vi "JYCalibrate.vi"(2 "error in (no error)":errorcluster, 3 "Actual Wavelength":dbl, 4 "JYMONOLib.IJYMonoReqd":refnum<k7>) -> (0 "error out":errorcluster, 1 "JYMONOLib.IJYMonoReqd 2":refnum<k7>)   [LabVIEW 2009]
doc: "JYCalibrate.vi\n\n\nInputs - MonoRefNum - LabView automation refnum for the mono\nUniqueID\n Actual Wavelength Remote - \n Error Cluster\n\nOutputs\n MonoRefNum - the LabView automation refnum for this mono\n is supplied as an output\n\n Error Cluster"
panel:
  out "UseUniqueID":bool
  in  "UniqueID":string
  in  "Mode Select":bool
  # "Local / Front Panel mode"
  # "Remote / Progarm mode"
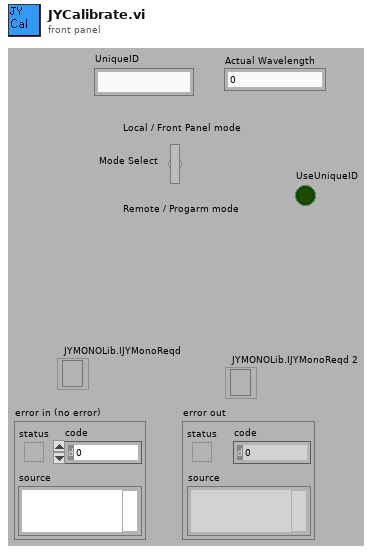
[diagram p1: front panel]
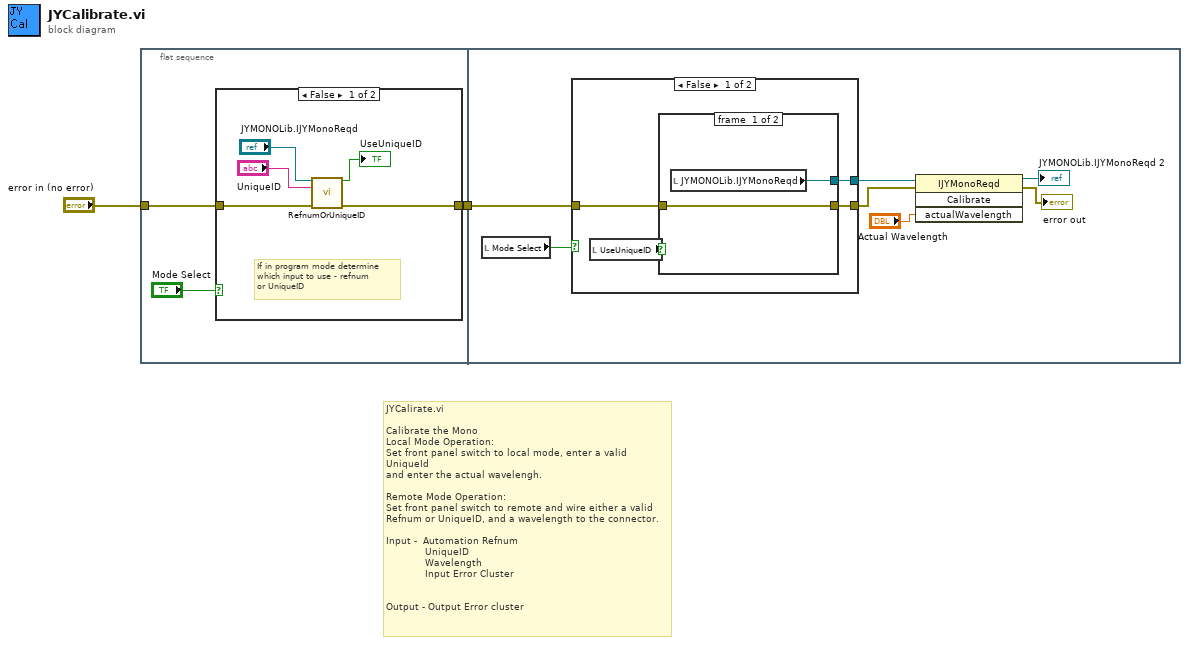
[diagram p0: block diagram]
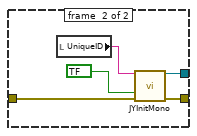
[diagram p3: hidden frame]
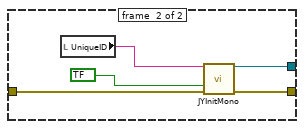
[diagram p4: hidden frame]
diagram:
  # "JYCalirate.vi\n\nCalibrate the Mono\nLocal Mode Operation:\nSet front panel switch to local mode, enter a valid UniqueId\nand enter the actual wavelengh.\n\nRemote Mode Operation:\nSet front panel switch to remote and wire either a valid\nRefnum or UniqueID, and a wavelength to the connector.\n\nInput -  Automation Refnum\n             UniqueID\n             Wavelength\n             Input Error Cluster\n\n\nOutput - Output Error cluster"
  n1 = flat-sequence {
    tunnel: "error in (no error)" -> [w4]
    tunnel: [w3] -> w1
    tunnel: w1 -> [w17]
    frame #0 {
      n2 = case shown="False" "Mode Select" {
        tunnel: w4 -> [w7 w11]
        tunnel: [w6 w11] -> w3
        frame #0 {
          # "If in program mode determine\nwhich input to use - refnum\nor UniqueID"
          n3 = call "RefnumOrUniqueID.vi"("Refnum IN"="JYMONOLib.IJYMonoReqd", "String in"="UniqueID", "error in (no error)"=w7) -> ("UseUniqueID"=→"UseUniqueID":bool, "error out"=w6:errorcluster)  [unwired: 11 out]
        }
        frame #1 {
        }
      }
    }
    frame #1 {
      n4 = local read "Mode Select"() -> (w18:bool)
      n5 = case shown="False" w18 {
        tunnel: w17 -> [w21 w34]
        tunnel: [w20 w31] -> w15
        tunnel: [w19 w30] -> w16
        frame #0 {
          n6 = local read "UseUniqueID"() -> (w22:bool)
          n7 = case shown="True" w22 {
            tunnel: w21 -> [w24 w27]
            tunnel: [w24 w26] -> w20
            tunnel: [w23 w25] -> w19
            frame #0 {
              n8 = local read "JYMONOLib.IJYMonoReqd"() -> (w23:refnum<k7>)
            }
            frame #1 {
              n9 = local read "UniqueID"() -> (w29:string)
              n10 = call "JYInitMono.vi"("Unique ID"=w29, "Force Init"=bool ?, "error in (no error)"=w27) -> ("Mono RefNum out"=w25:refnum<k7>, "error out"=w26:errorcluster)  [unwired: 1 in, 10 out]
            }
          }
        }
        frame #1 {
          n11 = local read "UniqueID"() -> (w33:string)
          n12 = call "JYInitMono.vi"("Unique ID"=w33, "Force Init"=bool ?, "error in (no error)"=w34) -> ("Mono RefNum out"=w30:refnum<k7>, "error out"=w31:errorcluster)  [unwired: 1 in, 10 out]
        }
      }
      n13 = invoke class="IJYMonoReqd" method="Calibrate"(reference=w16, error in=w15, "actualWavelength"="Actual Wavelength") -> (reference out=→"JYMONOLib.IJYMonoReqd 2":refnum<k7>, error out=→"error out":errorcluster)  [unwired: 1 in, 2 out]
    }
  }
